vi "Wire_Data.vi"(1 "待处理数据":u8[](array[numeric])) -> (0 "输出簇":T1)   [LabVIEW 2014]
panel:
  out "x*y 2":dbl
  out "x*y":dbl
  out "16位整型":u16
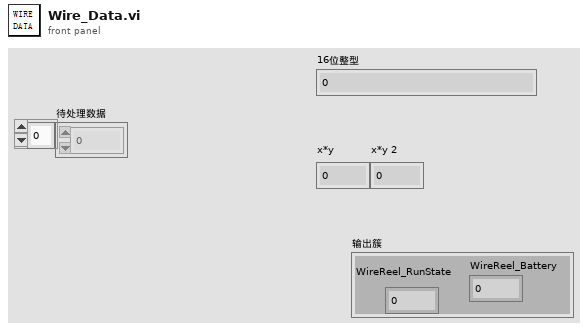
[diagram p1: front panel]
types:
  T1 = cluster{"WireReel_RunState\n":u8, "WireReel_Battery":dbl}
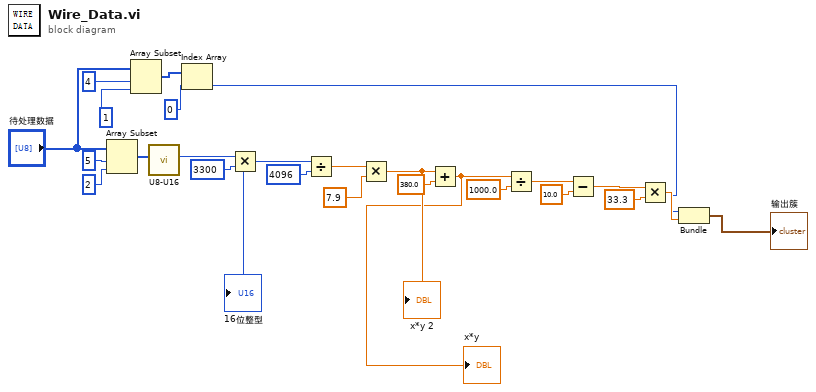
[diagram p0: block diagram]
diagram:
  n1 = Array Subset(array="待处理数据", index=5 ("索引"), length=2 ("索引")) -> (w8:u8[])
  n2 = Array Subset(array="待处理数据", index=4 ("长度（剩余）"), length=1 ("长度（剩余）")) -> (w3:u8[])
  n3 = call "U8-U16.vi"("数组"=w8) -> ("16位整型"=w24:u16)  [unwired: 8 in, 1 out]
  "16位整型" <- w24
  n4 = Index Array(array=w3, index=0 ("索引")) -> (element=w1:u8)
  n5 = Multiply(x=w24, y=3300) -> (x*y=w21:i32)
  n6 = Divide(x=w21, y=4096) -> (x/y=w19:dbl)
  n7 = Multiply(x=w19, y=7.9) -> (x*y=w18:dbl)
  "x*y 2" <- w18
  n8 = Add(x=w18, y=380.0) -> (x+y=w4:dbl)
  "x*y" <- w4
  n9 = Divide(x=w4, y=1000.0) -> (x/y=w15:dbl)
  n10 = Subtract(x=w15, y=10.0) -> (x-y=w13:dbl)
  n11 = Multiply(x=w13, y=33.3) -> (x*y=w11:dbl)
  n12 = Bundle(w1, w11) -> (→"输出簇":cluster{u8, dbl})  [unwired: 1 in]
